vi "Read Module Chuck.vi"(8 "error in":errorcluster, 10 "index":i32, 11 "WorkTable in":refnum<class "WorkTable Class.lvclass">) -> (0 "error out":errorcluster, 2 "Module Slots":T1[](array[typedef]), 3 "WorkTable out":refnum<class "WorkTable Class.lvclass">)   [LabVIEW 2011, in "WorkTable Class.lvclass"]
uses:
  WorkTable Class.lvclass
  Type Definitions/Worktable_Module Slot.ctl
  Vec3d Class/Vec3d Class.lvclass
  Orient3d Class/Orient3d Class.lvclass
  Utils/Type Definitions/Position_Orientation.ctl
  WorkTable Class.lvclass/WorkTable Class.ctl
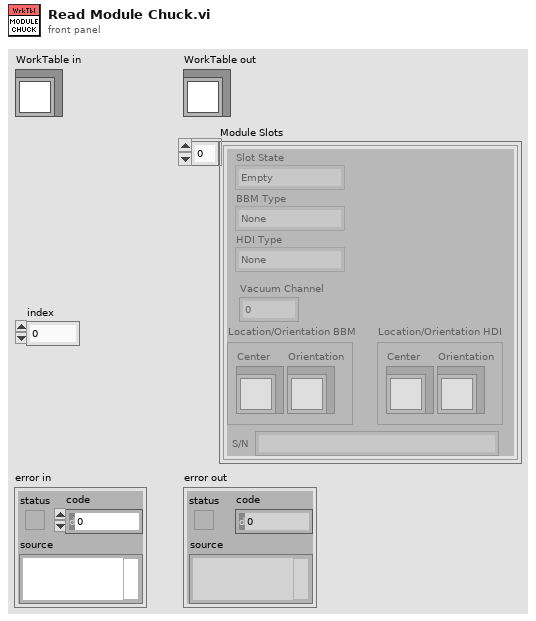
[diagram p1: front panel]
types:
  T1 = typedef "Worktable_Module Slot.ctl" = cluster{"Slot State":enum16{"Empty", "Bare HDI", "Unglued", "Stamped", "PartOnTop", "Weighted", "Unpotted", "Potted"}, "BBM Type":enum16{"None", "BBM", "GlassSlide"}, "HDI Type":enum16{"None", "HDI", "Polyimide"}, "Vacuum Channel":u8, "Location/Orientation BBM":T2, "Location/Orientation HDI":T2, "S/N":string}
  T2 = typedef "Position_Orientation.ctl" = cluster{"Center":refnum<class "Vec3d Class.lvclass">, "Orientation":refnum<class "Orient3d Class.lvclass">}
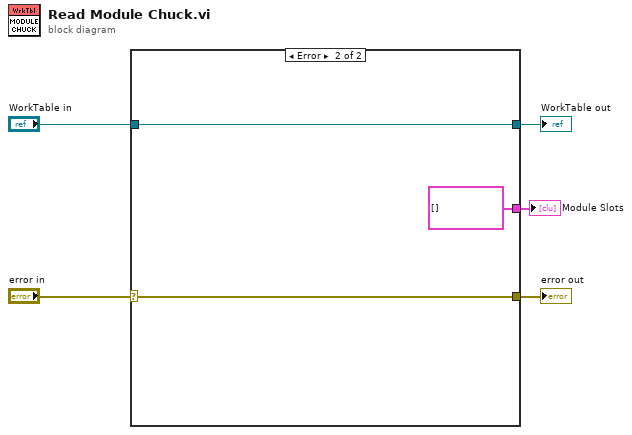
[diagram p0: block diagram]
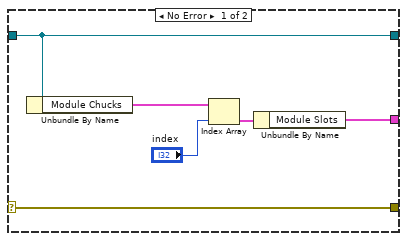
[diagram p2: hidden frame]
diagram:
  n1 = case shown="Error" "error in" {
    selector: "error in" -> [w11 w13]
    tunnel: [w11 w13] -> w4
    tunnel: [w10 w14] -> w2
    tunnel: "WorkTable in" -> [w10 w14]
    tunnel: [w6 T1[] [] ("Module Slots")] -> w1
    frame No Error {
      n2 = Unbundle By Name(w10) -> ("Module Chucks"=w9:cluster{"Module Slots":T1[]}[])
      n3 = Index Array(array=w9, index="index") -> (element=w7:cluster{"Module Slots":T1[]})
      n4 = Unbundle By Name(w7) -> ("Module Slots"=w6:T1[])
    }
    frame Error {
    }
  }
  "error out" <- w4
  "WorkTable out" <- w2
  "Module Slots" <- w1
